vi "KBDConnectJog.vi"() -> ()   [LabVIEW 2023]
uses:
  C:/Users/TSchofield/Downloads/Delete this/Thorlabs.MotionControl.KCube.BrushlessMotorCLI.dll
  Thorlabs.MotionControl.KCube.BrushlessMotorCLI.dll
  C:/Users/TSchofield/Downloads/Delete this/Thorlabs.MotionControl.Controls.dll
  Thorlabs.MotionControl.Controls.dll
panel:
  in  "stepSize":dbl
  in  "direction":i32(ring)=1 items=["Forward"=1, "Backward"=2]
  in  "SerialNumber":string
  in  "Disconnect":bool
  in  "Jog":bool
  out "Device Busy":bool
  out "Device Needs Homing":bool
  in  "KCubeBrushlessControl":refnum<k24>(container)
  # "Thorlabs Hardware: KBD - K-Cube Brushless DC Servo Driver\nhttps://www.thorlabs.com/thorproduct.cfm?partnumber=KBD101\n\nDescription: This VI will enable you to communicate with KBD101  to control  Brushless Stages & Actuators. The VI will first connect and initialize the device, home it, and await user command to move to a specified location.\n\nInstructions: \n1) Connect your KBD101  device to your PC & power the device, ensuring your stage/actutator is connected. For full device setup, the device product manual can be found on our website here. -https://www.thorlabs.com/thorproduct.cfm?partnumber=KBD101\n2) Enter the device serial number below.\n3) Ensure the device move path is clear for homing.\n4) Click 'Run' in the LabVIEW Toolbar which will attempt a connection, and send a home command in that order.\n5) Await for device to be be available, and to have finished homing.\n6) Input desired Jog Direction and step size position, and press 'Jog'.\n7) To end the Program click 'STOP'."
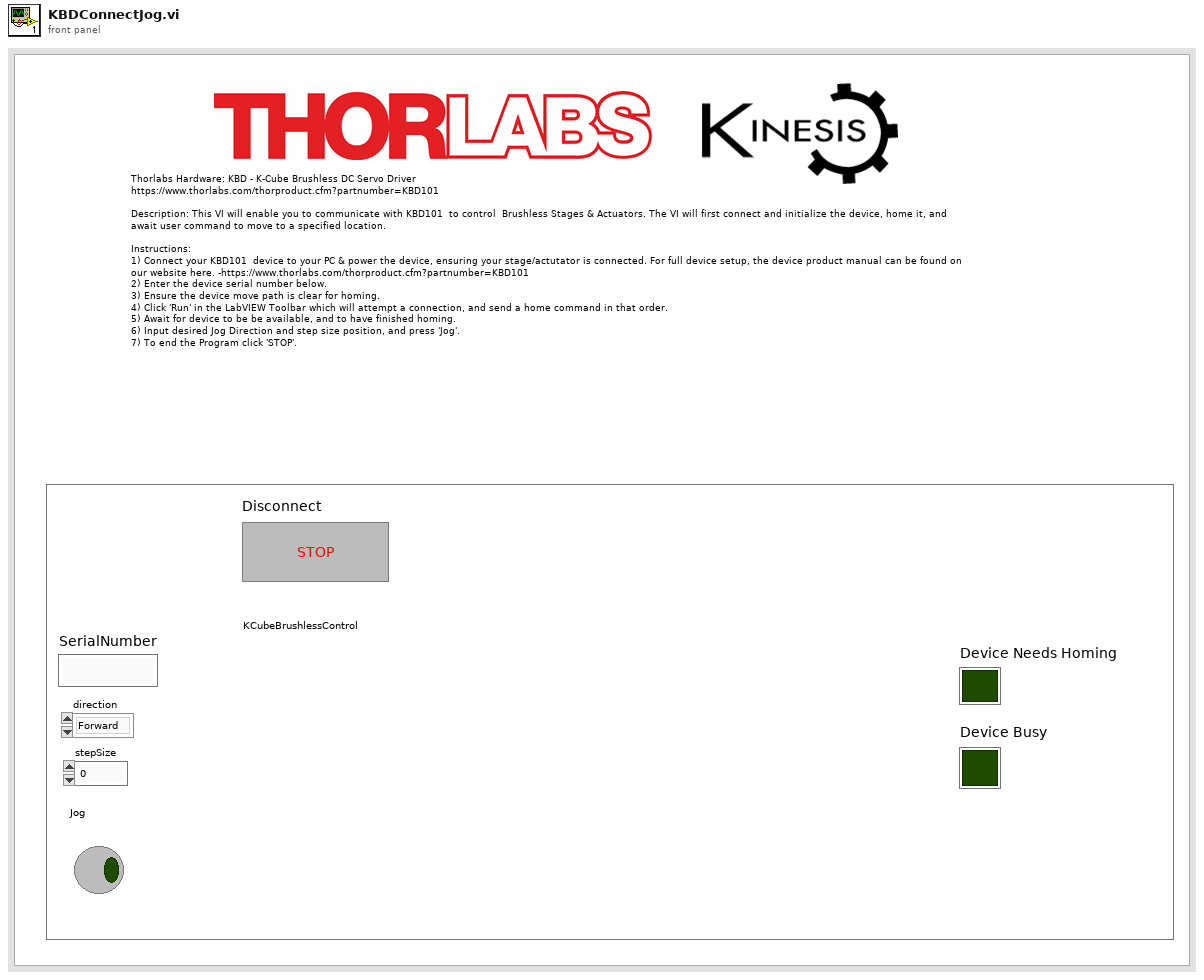
[diagram p1: front panel]
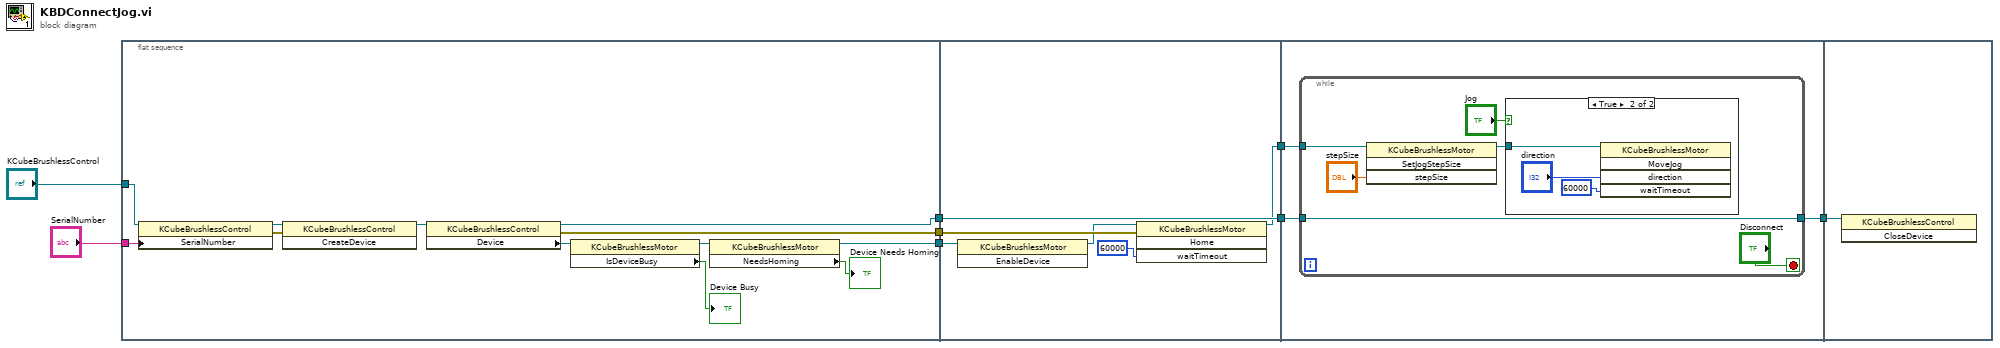
[diagram p0: block diagram]
diagram:
  n1 = flat-sequence {
    tunnel: "KCubeBrushlessControl" -> [w19]
    tunnel: "SerialNumber" -> [w17]
    tunnel: [w14] -> w8
    tunnel: [w13] -> w7
    tunnel: [w9] -> w2
    tunnel: w8 -> [w24]
    tunnel: w7 -> [w25]
    tunnel: [w25] -> w6
    tunnel: w2 -> [w23]
    tunnel: [w21] -> w1
    tunnel: w6 -> [w29]
    tunnel: [w28] -> w5
    tunnel: w1 -> [w27]
    tunnel: w5 -> [w39]
    frame #0 {
      n2 = property class="KCubeBrushlessControl"(reference=w19, "SerialNumber"=w17) -> (reference out=w20:refnum<k24>, error out=w18:errorcluster)  [unwired: 1 in]
      n3 = invoke class="KCubeBrushlessControl" method="CreateDevice"(reference=w20, error in=w18) -> (reference out=w16:refnum<k24>)  [unwired: 1 in, 2 out]
      n4 = property class="KCubeBrushlessControl"(reference=w16) -> (reference out=w13:refnum<k24>, error out=w14:errorcluster, "Device"=w11:refnum<k24>)  [unwired: 1 in]
      n5 = property class="KCubeBrushlessMotor"(reference=w11) -> (reference out=w10:refnum<k24>, "IsDeviceBusy"=→"Device Busy":bool)  [unwired: 1 in, 1 out]
      n6 = property class="KCubeBrushlessMotor"(reference=w10) -> (reference out=w9:refnum<k24>, "NeedsHoming"=→"Device Needs Homing":bool)  [unwired: 1 in, 1 out]
    }
    frame #1 {
      n7 = invoke class="KCubeBrushlessMotor" method="EnableDevice"(reference=w23) -> (reference out=w22:refnum<k24>)  [unwired: 2 in, 2 out]
      n8 = invoke class="KCubeBrushlessMotor" method="Home"(reference=w22, error in=w24, "waitTimeout"=60000) -> (reference out=w21:refnum<k24>)  [unwired: 1 in, 3 out]
    }
    frame #2 {
      n9 = while {
        tunnel: [w35] -> w28
        tunnel: w29 -> [w35]
        tunnel: w27 -> [w30]
        stop <- "Disconnect" stop-if-true
        n10 = invoke class="KCubeBrushlessMotor" method="SetJogStepSize"(reference=w30, "stepSize"="stepSize") -> (reference out=w31:refnum<k24>)  [unwired: 2 in, 3 out]
        n11 = case shown="True" "Jog" {
          tunnel: w31 -> [_ w36]
          frame False {
          }
          frame True {
            n12 = invoke class="KCubeBrushlessMotor" method="MoveJog"(reference=w36, "direction"="direction", "waitTimeout"=60000) -> ()  [unwired: 2 in, 5 out]
          }
        }
      }
    }
    frame #3 {
      n13 = invoke class="KCubeBrushlessControl" method="CloseDevice"(reference=w39) -> ()  [unwired: 2 in, 3 out]
    }
  }
